vi "CSM Check - State.vi"(8 "Matched Previous?":bool, 10 "Cross CSM Data (in)":T1={"Name(\"\" to use uuid)"="", "Current State"="", "Arguments"="", "Source Message"={"‘State"="", "’Arguments"="", "’Error"={"status"=FALSE, "code"=0, "source"=""}}, "Source Module"="", "Complete(T)/Start(F)"=FALSE, "LogType"=enum."State Change"}, 11 "GlobalLogFilter.lvclass":refnum<class "LogFilter.lvclass">) -> (0 "Matched? (dup)":bool, 2 "Cross CSM Data":T1={"Name(\"\" to use uuid)"="", "Current State"="", "Arguments"="", "Source Message"={"‘State"="", "’Arguments"="", "’Error"={"status"=FALSE, "code"=0, "source"=""}}, "Source Module"="", "Complete(T)/Start(F)"=FALSE, "LogType"=enum."State Change"}, 3 "GlobalLogFilter.lvclass (dup)":refnum<class "LogFilter.lvclass">)   [LabVIEW 2020, in "Communicable State Machine.lvlib" / "LogFilter.lvclass"]
uses:
  LogFilter.lvclass
  _CSM_GlobalLog_MSG.ctl
  _CSM_Response Source Message.ctl
  _CSM_GlobalLog_MSG_TYPE.ctl
  LogFilter.lvclass/LogFilter.ctl
  Communicable State Machine.lvlib
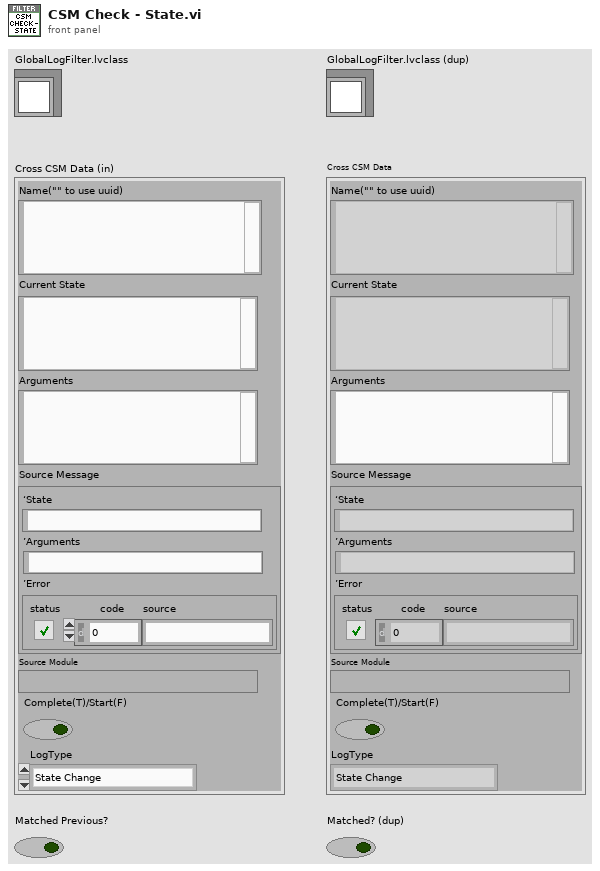
[diagram p1: front panel]
types:
  T1 = typedef "Communicable State Machine.lvlib/_CSM_GlobalLog_MSG.ctl" = cluster{"Name(\"\" to use uuid)":string, "Current State":string, "Arguments":string, "Source Message":T2, "Source Module":string, "Complete(T)/Start(F)":bool, "LogType":T3}
  T2 = typedef "Communicable State Machine.lvlib/_CSM_Response Source Message.ctl" = cluster{"‘State":string, "’Arguments":string, "’Error":errorcluster}
  T3 = typedef "Communicable State Machine.lvlib/_CSM_GlobalLog_MSG_TYPE.ctl" = enum16{"User Log", "State Change", "Status", "Interrupt", "Register", "Unregister", "Error Log", "Module Created", "Module Destroyed"}
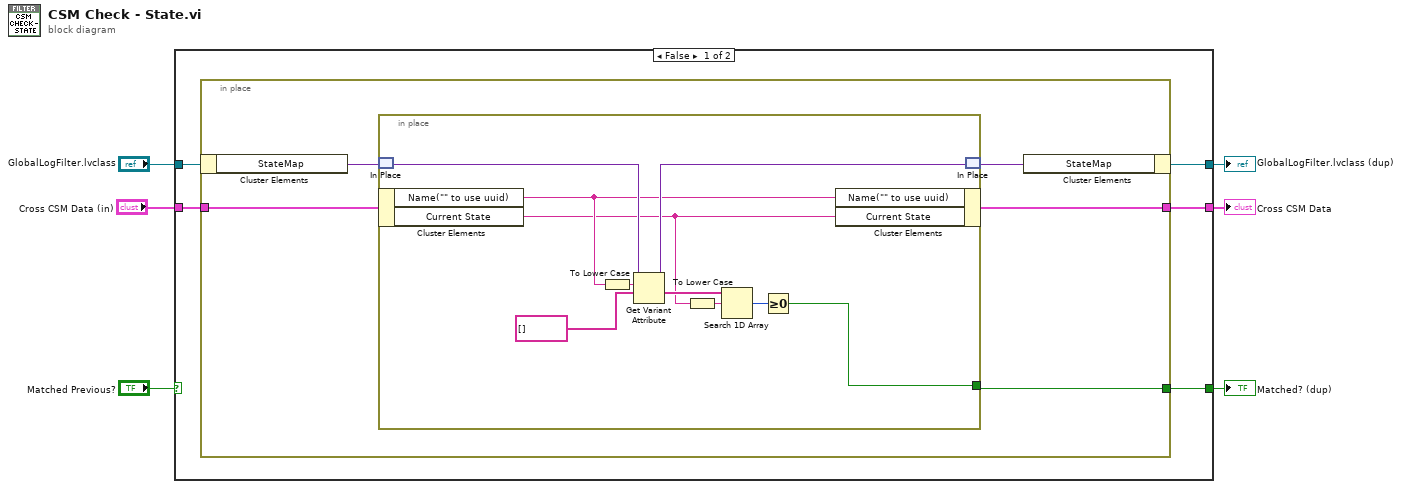
[diagram p0: block diagram]
diagram:
  n1 = case shown="False" "Matched Previous?" {
    selector: "Matched Previous?" -> [_ w28]
    tunnel: [w10 w29] -> w5
    tunnel: "Cross CSM Data (in)" -> [w11 w29]
    tunnel: [w9 w28] -> w3
    tunnel: [w7 w27] -> w2
    tunnel: "GlobalLogFilter.lvclass" -> [w8 w27]
    frame False {
      n2 = in-place {
        in-place-border: w11 -> [w16]
        in-place-border: [w15] -> w10
        in-place-border: [w14] -> w9
        n3 = in-place-cluster #1(w8) -> ("StateMap"=w13:variant)
        n4 = in-place {
          in-place-border: [w19] -> w14
          n5 = in-place-match #2(w13) -> (w26:variant)
          n6 = in-place-cluster #3(w16) -> ("Name(\"\" to use uuid)"=w24:string, "Current State"=w21:string)
          n7 = To Lower Case(string=w24) -> (all lower case string=w18:string)
          n8 = Get Variant Attribute(Variant=w26, name=w18, default value (empty Variant)=string[] []) -> (duplicate Variant=w25:variant, value=w22:string[])  [unwired: 1 in, 2 out]
          n9 = To Lower Case(string=w21) -> (all lower case string=w17:string)
          n10 = Search 1D Array(1D array=w22, element=w17) -> (index of element=w20:i32)  [unwired: 1 in]
          n11 = Greater Or Equal To 0?(x=w20) -> (x >= 0?=w19:bool)
          n12 = in-place-cluster #3("Name(\"\" to use uuid)"=w24, "Current State"=w21) -> (w15:T1)
          n13 = in-place-match #2(w25) -> (w12:variant)
        }
        n14 = in-place-cluster #1("StateMap"=w12) -> (w7:refnum<class "LogFilter.lvclass">)
      }
    }
    frame True {
    }
  }
  "Cross CSM Data" <- w5
  "Matched? (dup)" <- w3
  "GlobalLogFilter.lvclass (dup)" <- w2
